vi "Complex Multiply (SGL).vi"(8 "Input Valid":bool=TRUE, 10 "X2+j Y2":cluster{"Y2":fxp<+,32,32>, "X2":fxp<+,32,32>}, 11 "X1+j Y1":cluster{"Y1":fxp<+,32,32>, "X1":fxp<+,32,32>}) -> (0 "Output Valid":bool, 3 "Xout+j Yout":T1)   [LabVIEW 2011]
doc: "This VI performs single precsion complex multiply\n\n<b> Latency = 19 Ticks </b>"
types:
  T1 = cluster{"Yout":fxp<+,32,32>, "Xout":fxp<+,32,32>}
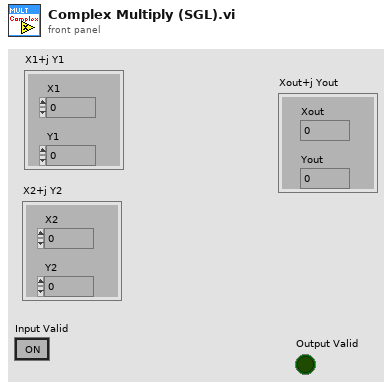
[diagram p1: front panel]
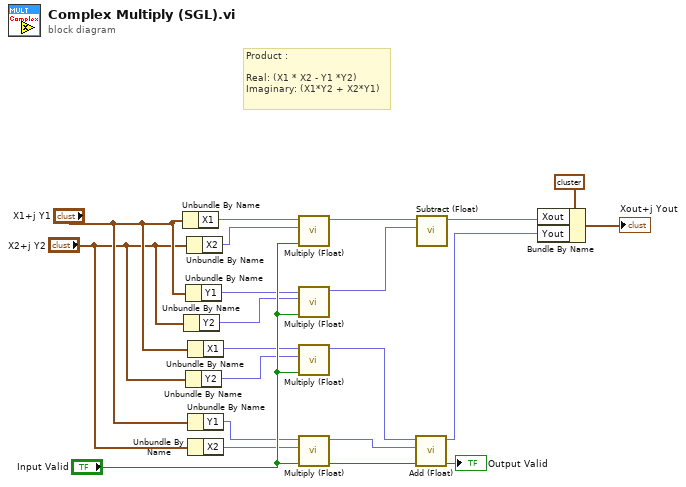
[diagram p0: block diagram]
diagram:
  # "Product :\n\nReal: (X1 * X2 - Y1 *Y2)\nImaginary: (X1*Y2 + X2*Y1)"
  n1 = Unbundle By Name("X1+j Y1") -> ("X1"=w9:fxp<+,32,32>)
  n2 = Unbundle By Name("X2+j Y2") -> ("Y2"=w7:fxp<+,32,32>)
  n3 = Unbundle By Name("X1+j Y1") -> ("Y1"=w8:fxp<+,32,32>)
  n4 = Unbundle By Name("X2+j Y2") -> ("Y2"=w5:fxp<+,32,32>)
  n5 = Unbundle By Name("X2+j Y2") -> ("X2"=w10:fxp<+,32,32>)
  n6 = Unbundle By Name("X1+j Y1") -> ("X1"=w6:fxp<+,32,32>)
  n7 = Unbundle By Name("X1+j Y1") -> ("Y1"=w2:fxp<+,32,32>)
  n8 = Unbundle By Name("X2+j Y2") -> ("X2"=w1:fxp<+,32,32>)
  n9 = call <userlib>:"Multiply (Float).vi"("Input Valid"="Input Valid", "b"=w10, "a"=w9) -> ("a*b"=w20:fxp<+,32,32>)  [unwired: 7 in, 1 out]
  n10 = call <userlib>:"Multiply (Float).vi"("Input Valid"="Input Valid", "b"=w7, "a"=w8) -> ("a*b"=w19:fxp<+,32,32>)  [unwired: 7 in, 1 out]
  n11 = call <userlib>:"Multiply (Float).vi"("Input Valid"="Input Valid", "b"=w5, "a"=w6) -> ("a*b"=w18:fxp<+,32,32>)  [unwired: 7 in, 1 out]
  n12 = call <userlib>:"Multiply (Float).vi"("Input Valid"="Input Valid", "b"=w1, "a"=w2) -> ("Output Valid"=w16:bool, "a*b"=w17:fxp<+,32,32>)  [unwired: 7 in]
  n13 = call <userlib>:"Add (Float).vi"("Input Valid"=w16, "b"=w17, "a"=w18) -> ("Output Valid"=→"Output Valid":bool, "a+b"=w12:fxp<+,32,32>)  [unwired: 7 in]
  n14 = call <userlib>:"Subtract (Float).vi"("b"=w19, "a"=w20) -> ("a-b"=w13:fxp<+,32,32>)  [unwired: 8 in, 1 out]
  n15 = Bundle By Name(cluster=T1 {"Yout"=0.0, "Xout"=0.0} ("Xout+j Yout"), "Xout"=w13, "Yout"=w12) -> (→"Xout+j Yout":T1)
